vi "Write Serial Data.vi"(7 "error in":errorcluster, 9 "SerialData":refnum<class "Data.lvclass">[](array[class]), 10 "binFile":refnum<file>) -> (0 "error out":errorcluster, 3 "binFileOut":refnum<file>)   [LabVIEW 2014, in "CRDS Data.lvclass"]
uses:
  CRDS Data.lvclass
  Data/Data.lvclass
  Devices/Alicat/Data/MC/AlicatMCData.lvclass
  crd_data_enum.ctl
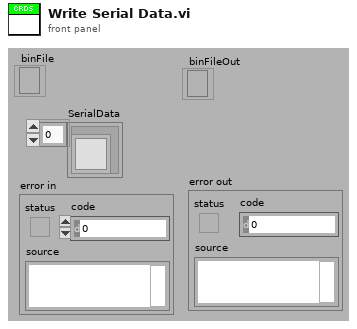
[diagram p1: front panel]
types:
  T1 = enum16{"big-endian, network order", "native, host order", "little-endian"}
  T2 = cluster{"P":sgl, "T":sgl, "Q":sgl, "Q0":sgl, "Qsp":sgl}
  T3 = typedef "crd_data_enum.ctl" = enum8{"Time", "RHw", "TRH", "P", "Tmean", "RHsense", "TQ", "PQ", "Q", "Q0", "Qcal", "Qset", "extDilFac", "taucorr", "tau0corr", "stdevtau", "ext", "extCorr", "etau", "tau", "tau0", "Purge_Data", "NoData", "reserved", "Ttec", "Ang Exp", "Gamma", "filter", "fOverride", "notes", "max amp", "Tthermistor", "RhdilFac", "Psense", "TRHsense_bank", "RHsense_bank", "MFC_Data", "Thum", "ThumSP", "O3 Flow", "Pinlet Flow", "CLAP Flow", "O3 Add Valve", "O2 Valve", "O3 Cal"}
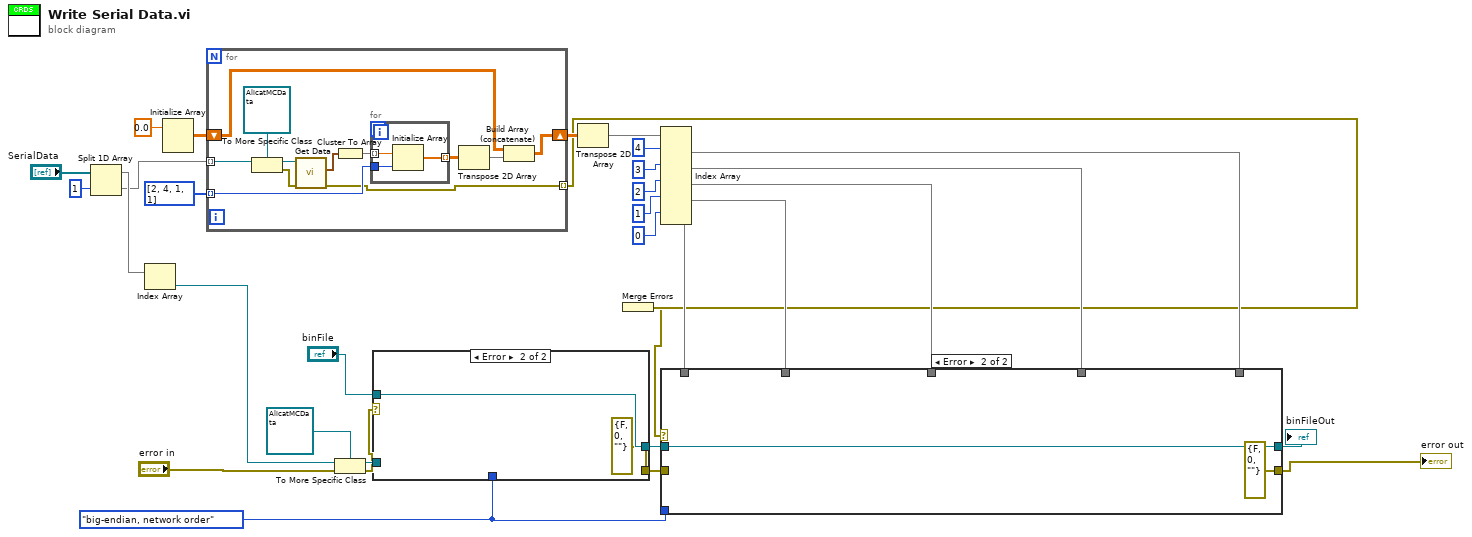
[diagram p0: block diagram]
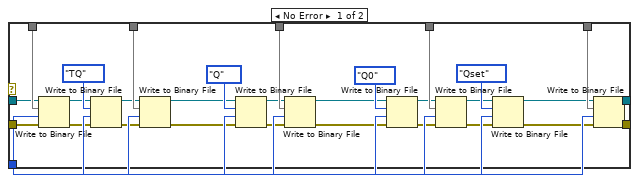
[diagram p2: hidden frame]
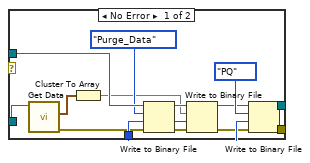
[diagram p3: hidden frame]
diagram:
  w19 = T1."big-endian, network order" ("byte order (0:big-endian, network order)")
  n1 = Split 1D Array(array="SerialData", index=1) -> (first subarray=w11:refnum<class "Data.lvclass">[], second subarray=w8:refnum<class "Data.lvclass">[])
  n2 = Index Array(array=w11) -> (element=w9:refnum<class "Data.lvclass">)  [unwired: 1 in]
  n3 = Initialize Array(sgl 0.0 ("element")) -> (w28:sgl[][])  [unwired: 2 in]
  n4 = for {
    tunnel: w8 -> [w41] mode=indexing
    tunnel: i32[] [2, 4, 1, 1] -> [w38] mode=indexing
    shift-right: [w34] -> w27
    shift-left: w28 -> [w35]
    tunnel: [w33] -> w7 mode=indexing
    n5 = To More Specific Class(target class=refnum<class "AlicatMCData.lvclass"> refnum ("Alicat.lvlib:AlicatMCData.lvclass"), reference=w41) -> (specific class reference=w43:refnum<class "AlicatMCData.lvclass">, error out=w42:errorcluster)  [unwired: 1 in]
    n6 = call "Get Data.vi"("error in"=w42, "AlicatMData in"=w43) -> ("error out"=w33:errorcluster, "SystemData"=w40:T2)  [unwired: 7 in, 1 out]
    n7 = Cluster To Array(cluster=w40) -> (array=w39:sgl[])
    n8 = for {
      tunnel: w39 -> [w47] mode=indexing
      tunnel: w38 -> [w46]
      tunnel: [w45] -> w37 mode=indexing
      n9 = Initialize Array(w47, w46) -> (w45:sgl[])
    }
    n10 = Transpose 2D Array(2D array=w37) -> (transposed array=w36:sgl[][])
    n11 = Build Array (concatenate)(w35, w36) -> (w34:sgl[][])
  }
  n12 = To More Specific Class(target class=refnum<class "AlicatMCData.lvclass"> refnum ("Alicat.lvlib:AlicatMCData.lvclass"), reference=w9, error in="error in") -> (specific class reference=w32:refnum<class "AlicatMCData.lvclass">, error out=w3:errorcluster)
  n13 = case shown="Error" w3 {
    tunnel: w32 -> [w61 _]
    tunnel: w19 -> [w60 _]
    tunnel: "binFile" -> [w59 w63]
    tunnel: [w56 errorcluster {"status"=FALSE, "code"=0, "source"=""} ("error out")] -> w5
    tunnel: [w55 w63] -> w4
    frame No Error {
      n14 = call "Get Data.vi"("AlicatMData in"=w61) -> ("error out"=w52:errorcluster, "SystemData"=w51:T2)  [unwired: 8 in, 1 out]
      n15 = Cluster To Array(cluster=w51) -> (array=w50:sgl[])
      n16 = Write to Binary File(file (use dialog)=w59, data=crd_data_enum."Purge_Data" ("CRD_Data_Enum"), error in=w52, 9:w60) -> (refnum out=w58:refnum<file>, error out=w53:errorcluster)  [unwired: 2 in, 1 out]
      n17 = Write to Binary File(file (use dialog)=w58, data=w50, error in=w53, 9:w60) -> (refnum out=w49:refnum<file>, error out=w48:errorcluster)  [unwired: 2 in, 1 out]
      n18 = Write to Binary File(file (use dialog)=w49, data=crd_data_enum."PQ" ("CRD_Data_Enum"), error in=w48, 9:w60) -> (refnum out=w55:refnum<file>, error out=w56:errorcluster)  [unwired: 2 in, 1 out]
    }
    frame Error {
    }
  }
  n19 = Transpose 2D Array(2D array=w27) -> (transposed array=w26:sgl[][])
  n20 = Merge Errors(w7) -> (w2:errorcluster)
  n21 = Index Array(array=w26, index (row) #1=4 ("index (row)"), index (row) #2=3 ("index (row)"), index (row) #3=2 ("index (row)"), index (row) #4=1 ("index (row)"), index (row) #5=0 ("index (row)")) -> (element #1=w15:sgl[], element #2=w16:sgl[], element #3=w20:sgl[], element #4=w17:sgl[], element #5=w18:sgl[])  [unwired: 5 in]
  n22 = case shown="Error" w2 {
    tunnel: w20 -> [w93 _]
    tunnel: w19 -> [w92 _]
    tunnel: w18 -> [w91 _]
    tunnel: w17 -> [w90 _]
    tunnel: w16 -> [w89 _]
    tunnel: w15 -> [w88 _]
    tunnel: [w87 w95] -> w14
    tunnel: [w86 errorcluster {"status"=FALSE, "code"=0, "source"=""} ("error out")] -> w1
    tunnel: w5 -> [w85 _]
    tunnel: w4 -> [w84 w95]
    frame No Error {
      n23 = Write to Binary File(file (use dialog)=w84, data=w91, error in=w85, 9:w92) -> (refnum out=w80:refnum<file>, error out=w79:errorcluster)  [unwired: 2 in, 1 out]
      n24 = Write to Binary File(file (use dialog)=w80, data=crd_data_enum."TQ" ("CRD_Data_Enum"), error in=w79, 9:w92) -> (refnum out=w83:refnum<file>, error out=w82:errorcluster)  [unwired: 2 in, 1 out]
      n25 = Write to Binary File(file (use dialog)=w83, data=w90, error in=w82, 9:w92) -> (refnum out=w75:refnum<file>, error out=w74:errorcluster)  [unwired: 2 in, 1 out]
      n26 = Write to Binary File(file (use dialog)=w75, data=crd_data_enum."Q" ("CRD_Data_Enum"), error in=w74, 9:w92) -> (refnum out=w77:refnum<file>, error out=w78:errorcluster)  [unwired: 2 in, 1 out]
      n27 = Write to Binary File(file (use dialog)=w77, data=w93, error in=w78, 9:w92) -> (refnum out=w70:refnum<file>, error out=w69:errorcluster)  [unwired: 2 in, 1 out]
      n28 = Write to Binary File(file (use dialog)=w70, data=crd_data_enum."Q0" ("CRD_Data_Enum"), error in=w69, 9:w92) -> (refnum out=w73:refnum<file>, error out=w72:errorcluster)  [unwired: 2 in, 1 out]
      n29 = Write to Binary File(file (use dialog)=w73, data=w89, error in=w72, 9:w92) -> (refnum out=w65:refnum<file>, error out=w64:errorcluster)  [unwired: 2 in, 1 out]
      n30 = Write to Binary File(file (use dialog)=w65, data=crd_data_enum."Qset" ("CRD_Data_Enum"), error in=w64, 9:w92) -> (refnum out=w67:refnum<file>, error out=w68:errorcluster)  [unwired: 2 in, 1 out]
      n31 = Write to Binary File(file (use dialog)=w67, data=w88, error in=w68, 9:w92) -> (refnum out=w87:refnum<file>, error out=w86:errorcluster)  [unwired: 2 in, 1 out]
    }
    frame Error {
    }
  }
  "error out" <- w1
  "binFileOut" <- w14
